vi "Authorization.vi"() -> (0 "Authorization":string[](array[string]))   [LabVIEW 2020]
uses:
  Global.vi
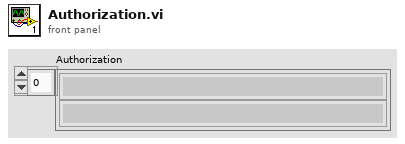
[diagram p1: front panel]
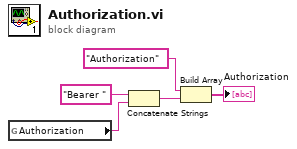
[diagram p0: block diagram]
diagram:
  n1 = global read "Global.vi" "Authorization"() -> (w3:string)
  n2 = Concatenate Strings("Bearer ", w3) -> (w2:string)
  n3 = Build Array("Authorization", w2) -> (→"Authorization":string[])
